vi "Relays - Synchronized.vi"() -> ()   [LabVIEW 2017]
uses:
  <vilib>/Platform/TimedLoop/XDataNode/wakeup.ctl
  <vilib>/Platform/TimedLoop/XDataNode/XDNodeRunTimeDep.lvlib
  <vilib>/Platform/TimedLoop/XDataNode/nitl_modes.ctl
  <vilib>/Platform/TimedLoop/XDataNode/timing_clust.ctl
  <vilib>/Platform/TimedLoop/XDataNode/XDataNode.xnode
  <vilib>/DAQmx/create/timing.llb/DAQmx Create Timing Source (Digital Edge using Counter).vi
panel:
  out "error out":errorcluster
  in  "error in":errorcluster
  in  "Pulse Length":dbl[unit]
  in  "Switch Time":dbl[unit]
  in  "Stop":bool
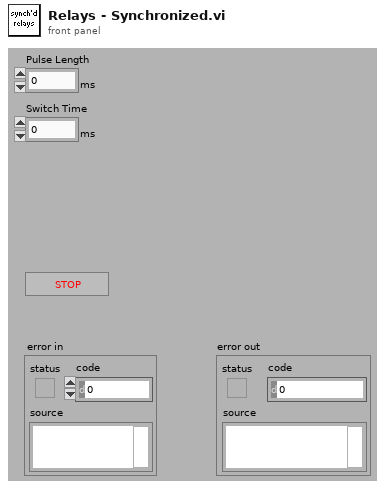
[diagram p1: front panel]
types:
  T1 = typedef "XDNodeRunTimeDep.lvlib/timing_clust.ctl" = cluster{"Expected End [f-1]":u64, "Actual End [f-1]":u64, "Finished Late? [f-1]":bool, "Expected End [i-1]":u64, "Actual End [i-1]":u64, "Finished Late? [i-1]":bool, "Expected Start [i]":u64, "Actual Start [i]":u64, "Expected Start [f]":u64, "Actual Start [f]":u64, "Source Name":string, "Structure Name":string, "Period":i64, "Deadline":i64, "Offset":i64, "Start":i64, "Priority":i32, "Timeout":i32, "Mode":T2, "Wakeup Reason":T3, "Error":errorcluster, "Source Type":string, "Secondary Source Type":string, "Global End Time":u64, "Global Start Time":u64, "Frame Duration":u64, "Iteration Duration":u64, "Assigned CPU":i32, "I/O Scan Engine Mode":u32}
  T2 = typedef "XDNodeRunTimeDep.lvlib/nitl_modes.ctl" = enum32{"No Change", "Process missed periods, maintain original phase", "Discard missed periods, maintain original phase", "Process missed periods, ignore original phase", "Discard missed periods, ignore original phase"}
  T3 = typedef "XDNodeRunTimeDep.lvlib/wakeup.ctl" = enum32{"Normal", "Aborted", "Asynchronous wakeup", "Timing source error", "Timed loop error", "Timeout"}
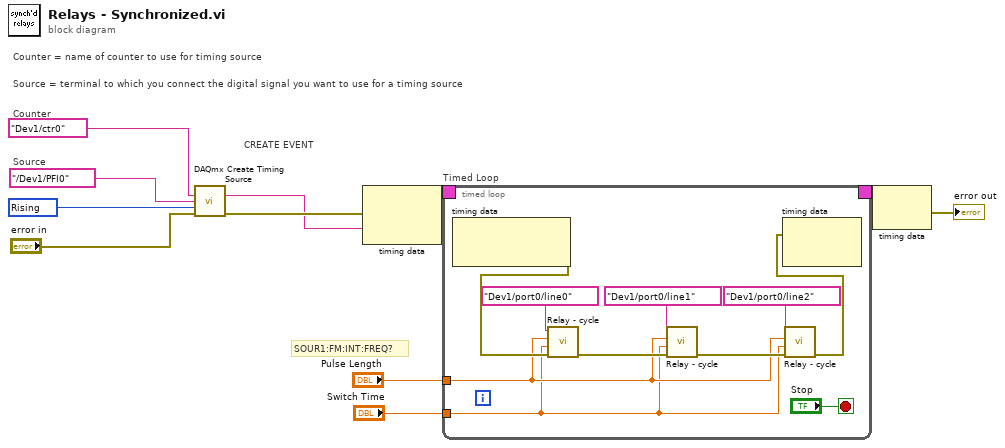
[diagram p0: block diagram]
diagram:
  w5 = 10280 items=["Rising"=10280, "Falling"=10171] ("edge")
  # "SOUR1:FM:INT:FREQ?"
  # "CREATE EVENT"
  # "Counter = name of counter to use for timing source"
  # "Counter"
  # "Source"
  # "Source = terminal to which you connect the digital signal you want to use for a timing source"
  n1 = call-poly <vilib>:"DAQmx Create Timing Source.vi"("counter"=tag "Dev1/ctr0", "source"=tag "/Dev1/PFI0", "edge"=w5, "error in"="error in") -> ("timing source out"=w8:string, "error out"=w9:errorcluster)  [unwired: 2 in, 8 out]
  n2 = node-c288(w9, w8) -> (w11:T1)
  n3 = timed-loop "Timed Loop" {
    timing-out: [_] -> w10
    timing: w11 -> [_]
    tunnel: "Switch Time" -> [w12]
    tunnel: "Pulse Length" -> [w13]
    stop <- "Stop" stop-if-true
    n4 = node-c288() -> (w14:errorcluster)  [unwired: 2 out]
    n5 = call "Relay - cycle.vi"("error in"=w14, "switch time"=w12, "pulse length"=w13, "task in"=tag "Dev1/port0/line0") -> ("error out"=w17:errorcluster)  [unwired: 7 out]
    n6 = call "Relay - cycle.vi"("error in"=w17, "switch time"=w12, "pulse length"=w13, "task in"=tag "Dev1/port0/line1") -> ("error out"=w16:errorcluster)  [unwired: 7 out]
    n7 = call "Relay - cycle.vi"("error in"=w16, "switch time"=w12, "pulse length"=w13, "task in"=tag "Dev1/port0/line2") -> ("error out"=w15:errorcluster)  [unwired: 7 out]
    n8 = node-c288(w15) -> ()  [unwired: 2 out]
  }
  n9 = node-c288(w10) -> (→"error out":errorcluster)
